vi "FXP_Nbar_Re_Kx.vi"(7 "ref":fxp<+/-,32,5>, 8 "NS":u8=9, 10 "Nbar":fxp<+/-,32,5>) -> (2 "del u_x":fxp<+/-,32,16>)   [LabVIEW 2019]
doc: "Given an input array X and a reference to a memory item, comput the dot product,\neg K.*X. X can be a vector up to length = 9.\n\nND is the size of the vectors.\n\n\nTHIS VI IS DIFFERENT FROM \"SGL_K2_times_xd\" by different sizes allowed."
uses:
  <vilib>/Platform/TimedLoop/XDataNode/timing_clust.ctl
  <vilib>/Platform/TimedLoop/XDataNode/nitl_modes.ctl
  <vilib>/Platform/TimedLoop/XDataNode/wakeup.ctl
  typeDefs/Kz_bram.ctl
  typeDefs/x_vec_bram.ctl
  <vilib>/rvi/IPIntegrationNode/IPINode_Typedef/niFpgaIPINodeSupportedFamilies.ctl
  <vilib>/Utility/error.llb/Clear Errors.vi
  <vilib>/rvi/Emulation/niFpgaSctlEmulationGetInTimedLoop.vi
  <vilib>/rvi/Emulation/niFpgaEmulationIsFPGAContextNoSignature.vi
  <vilib>/rvi/DataTransferAndStorage/Container/Common/niFpgaContainerGetUniqueNameForEmu.vi
  <vilib>/rvi/Memory/Memory_Emulation/niFpgaMemoryEmulationCacheClearOnFirstRun.vi
  <vilib>/rvi/Memory/Memory_Emulation/nirvimemoryEmulationManagerCache_MakeExclusive.vi
  <vilib>/rvi/Memory/Memory_Emulation/niFpgaMemoryEmulationValidateCache.vi
  <vilib>/rvi/Memory/Memory_Emulation/nirvimemoryEmulationManagerCache_InsertValue.vi
  <vilib>/rvi/Memory/Memory_Emulation/nirvimemoryEmulationManagerCache_ReleaseExclusive.vi
  <vilib>/rvi/Memory/Memory_Emulation/nirvimemoryEmulationManagerCache_GetValue.vi
  <vilib>/rvi/Memory/Memory_Emulation/nirvimemoryEmulationManagerCache_SetValue.vi
  <vilib>/rvi/Emulation/niFpgaProcessEmulError.vi
  <vilib>/rvi/DataTransferAndStorage/Container/Common/niFpgaContainerExecOnDevCompGetState.vi
  <vilib>/rvi/errors/nirviReportUnexpectedCaseInternalError (U32).vi
  <vilib>/rvi/Emulation/niFpgaSctlEmulationResourceMgr.vi
  <vilib>/rvi/IPIntegrationNode/IPINode_Utilities/niFpgaIPINodeSimCore.vi
  <vilib>/Platform/TimedLoop/XDataNode/XDataNode.xnode
  <vilib>/rvi/DataTransferAndStorage/Container/XNode/niFpgaContainer.xnode
  <vilib>/rvi/DataTransferAndStorage/Register/Emulation/niFpgaRegisterEmulation.vi
  <vilib>/rvi/Memory/Memory_Emulation/niFpgaMemoryEmulationRefIn.vi
  <vilib>/rvi/FXPMathLib/FxpSub/XNode/nifxpmath_Sub.xnode
  <vilib>/rvi/XilinxIP/XIPIN_XNode/niFpgaXIPIN.xnode
  dspAccumulators/MAC_32-15_by_32-5/Multiply_Accumulator_D8DE52605E734182ABB00CFADECE4F1B.dll
  <vilib>/rvi/IPIntegrationNode/IPINode_Xnode/niFpgaIPINode.xnode
  <vilib>/Platform/TimedLoop/XDataNode/XDNodeRunTimeDep.lvlib
  <vilib>/rvi/FXPMathLib/sim/FxpSim.dll
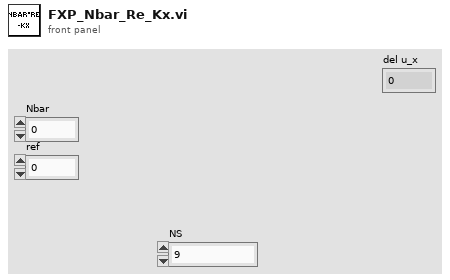
[diagram p1: front panel]
types:
  T1 = typedef "XDNodeRunTimeDep.lvlib/timing_clust.ctl" = cluster{"Expected End [f-1]":u64, "Actual End [f-1]":u64, "Finished Late? [f-1]":bool, "Expected End [i-1]":u64, "Actual End [i-1]":u64, "Finished Late? [i-1]":bool, "Expected Start [i]":u64, "Actual Start [i]":u64, "Expected Start [f]":u64, "Actual Start [f]":u64, "Source Name":string, "Structure Name":string, "Period":i64, "Deadline":i64, "Offset":i64, "Start":i64, "Priority":i32, "Timeout":i32, "Mode":T2, "Wakeup Reason":T3, "Error":errorcluster, "Source Type":string, "Secondary Source Type":string, "Global End Time":u64, "Global Start Time":u64, "Frame Duration":u64, "Iteration Duration":u64, "Assigned CPU":i32, "I/O Scan Engine Mode":u32}
  T2 = typedef "XDNodeRunTimeDep.lvlib/nitl_modes.ctl" = enum32{"No Change", "Process missed periods, maintain original phase", "Discard missed periods, maintain original phase", "Process missed periods, ignore original phase", "Discard missed periods, ignore original phase"}
  T3 = typedef "XDNodeRunTimeDep.lvlib/wakeup.ctl" = enum32{"Normal", "Aborted", "Asynchronous wakeup", "Timing source error", "Timed loop error", "Timeout"}
  T4 = typedef "x_vec_bram.ctl" = refnum<k21>
  T5 = typedef "Kz_bram.ctl" = refnum<k21>
  T6 = typedef "niFpgaIPINodeSupportedFamilies.ctl" = cluster{"unlimited?":bool, "supported targets":string[]}
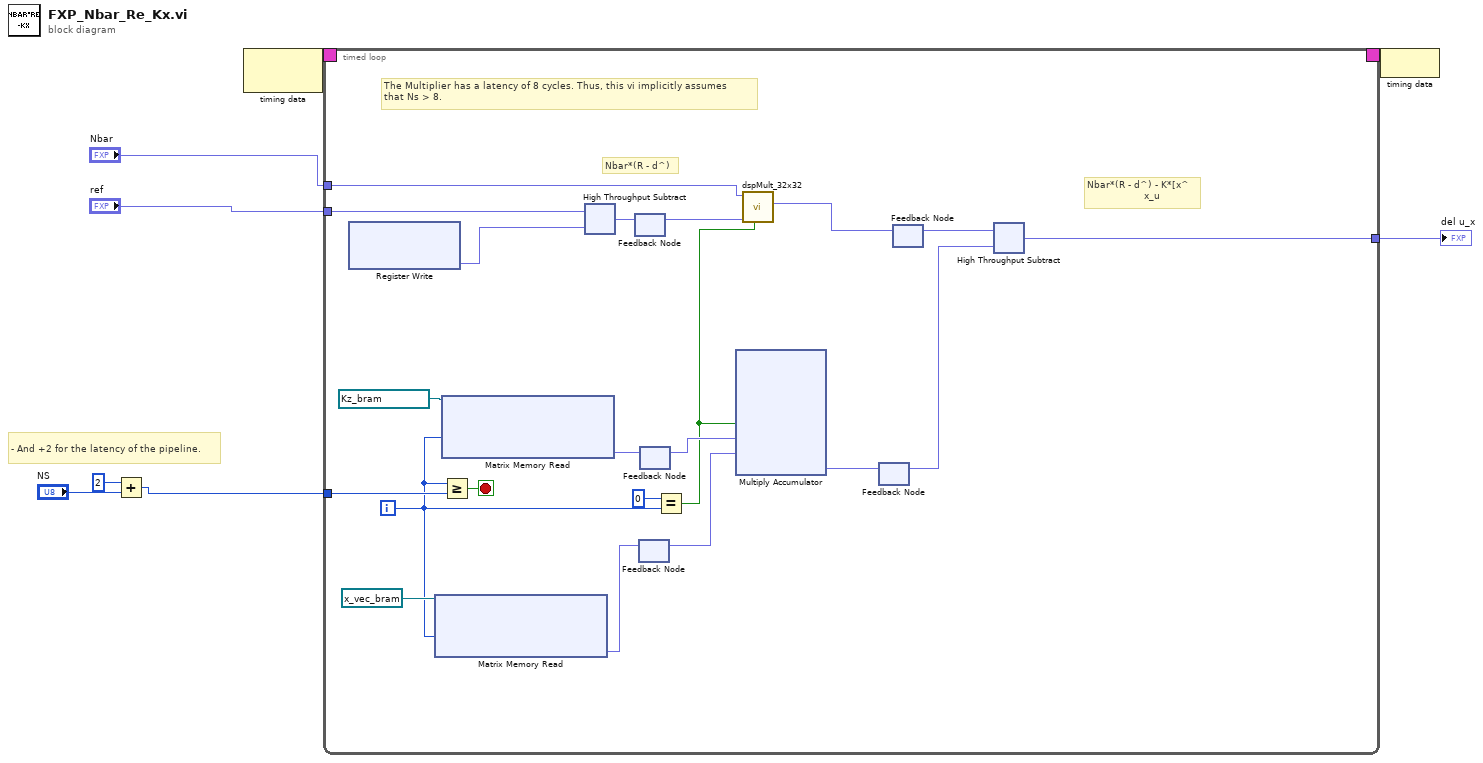
[diagram p0: block diagram]
diagram:
  # "- And +2 for the latency of the pipeline."
  n1 = Add(x=u8 2, y="NS") -> (x+y=w5:u8)
  n2 = node-c288() -> (w8:T1)  [unwired: 1 in]
  n3 = timed-loop {
    timing: w8 -> [_]
    timing-out: [_] -> w7
    tunnel: w5 -> [w28]
    tunnel: [w17] -> w3
    tunnel: "ref" -> [w20]
    tunnel: "Nbar" -> [w11]
    i -> [w15]
    stop <- w29 stop-if-true
    # "The Multiplier has a latency of 8 cycles. Thus, this vi implicitly assumes\nthat Ns > 8."
    # "Nbar*(R - d^) - K*[x^\n                   x_u"
    # "Nbar*(R - d^)"
    n4 = xnode "Register Write"() -> ("Data"=w9:fxp<+/-,32,6>)  [unwired: 1 in, 1 out]
    n5 = xnode "Matrix Memory Read"("Address"=w15, "Memory In"=T4 "xk_0_2" ("Memory")) -> ("Data"=w14:fxp<+/-,32,6>)  [unwired: 1 out]
    n6 = xnode "Matrix Memory Read"("Address"=w15, "Memory In"=T5 "K_FXP_row1" ("Memory")) -> ("Data"=w26:fxp<+/-,32,10>)  [unwired: 1 out]
    n7 = Greater Or Equal?(x=w15, y=w28) -> (x >= y?=w29:bool)
    n8 = xnode "High Throughput Subtract"("x"=w20, "y"=w9) -> ("x-y"=w21:fxp<+/-,32,5>)
    n9 = feedback #1() -> (w12:fxp<+/-,32,5>)  [unwired: 1 in]
    n10 = feedback-in #1(w21) -> ()
    n11 = feedback #2() -> (w25:fxp<+/-,32,6>)  [unwired: 1 in]
    n12 = feedback-in #2(w14) -> ()
    n13 = feedback-in #3(w26) -> ()
    n14 = feedback #3() -> (w23:fxp<+/-,32,10>)  [unwired: 1 in]
    n15 = Equal?(x=0, y=w15) -> (x = y?=w13:bool)
    n16 = xnode ("Multiply Accumulator")("sclr"=w13, "a"=w23, "b"=w25) -> ("s"=w24:fxp<+/-,32,16>)  [unwired: 1 in]
    n17 = call "dspMult_32x32.vi"("sclr"=w13, "b"=w12, "a"=w11) -> ("p"=w10:fxp<+/-,64,10>)  [unwired: 8 in]
    n18 = feedback #4() -> (w18:fxp<+/-,32,16>)  [unwired: 1 in]
    n19 = feedback-in #4(w24) -> ()
    n20 = feedback #5() -> (w19:fxp<+/-,64,10>)  [unwired: 1 in]
    n21 = feedback-in #5(w10) -> ()
    n22 = xnode "High Throughput Subtract"("x"=w19, "y"=w18) -> ("x-y"=w17:fxp<+/-,32,5>)
  }
  "del u_x" <- w3
  n23 = node-c288(w7) -> ()
